vi "All Verifies With Labels.vi"   [LabVIEW 2020, in "Caraya Extension Tests.lvclass"]
uses:
  Caraya Extension Tests.lvclass
  Source/Approval Tests/Options/Options.lvclass/Options.ctl
  Source/Approval Tests/Naming Data/Naming Data.lvclass/Naming Data.ctl
  Source/Approval Tests/Options/Options.lvclass
  Source/Approval Tests/Scrubber/Scrubber.lvclass
  Source/Approval Tests/Namer/Namer.lvclass
  Source/Approval Tests/Naming Data/Naming Data.lvclass
  Source/Approval Tests/Reporter/Reporter.lvclass
  Source/Approval Tests/Text Comparator/Text Comparator.lvclass
  870c6c77-fc99-4cce-8b97-a4330b55fadd.vi
  Source/Extensions/Caraya.Extension/Caraya.Extension.lvlib
  <vilib>/addons/_JKI Toolkits/Caraya/classes/Test/Test.lvclass
  f52be7d2-abca-4f6a-8aa8-cd22b4bd47f7.vi
  9461663a-62e6-4c7f-8db7-86399d0571fe.vi
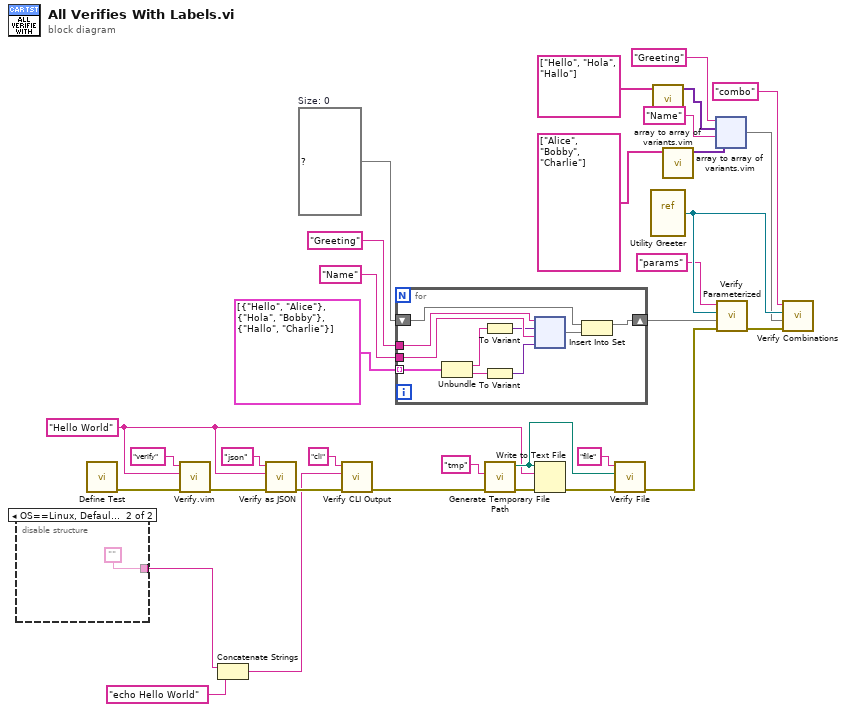
[diagram p0: block diagram]
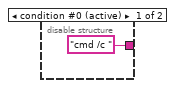
[diagram p2: hidden frame]
diagram:
  w24 = set{map{string, variant}} {}  # Size: 0
  w8 = "Hello World"
  n1 = disable-structure shown="OS==Linux, Default" {
    disable-tunnel: ["cmd /c " ""] -> w5
    frame condition #0 (active) {
    }
    frame condition #1 {
    }
  }
  n2 = call <vilib>:"Define Test.vi"() -> ("error out"=w31:errorcluster)  [unwired: 10 in, 1 out]
  n3 = call "Verify.vim"("error in"=w31, "Test Data"=w8, "Label"="verify") -> ("error out"=w33:errorcluster)  [unwired: 7 in, 1 out]
  n4 = Concatenate Strings(w5, "echo Hello World" ("string")) -> (w6:string)
  n5 = call "Verify as JSON.vi"("error in"=w33, "Anything"=w8, "Label"="json") -> ("error out"=w32:errorcluster)  [unwired: 7 in, 1 out]
  n6 = call "Verify CLI Output.vi"("error in"=w32, "command line"=w6, "Label"="cli") -> ("error out"=w28:errorcluster)  [unwired: 7 in, 1 out]
  n7 = for {
    tunnel: "Greeting" -> [w45]
    tunnel: cluster{string, string}[] [{"Hello", "Alice"}, {"Hola", "Bobby"}, {"Hallo", "Charlie"}] -> [w43] mode=indexing
    tunnel: "Name" -> [w44]
    shift-right: [w37] -> w25
    shift-left: w24 -> [w36]
    n8 = Unbundle(w43) -> (w42:string, w41:string)
    n9 = To Variant(anything=w42) -> (Variant=w39:variant)
    n10 = To Variant(anything=w41) -> (Variant=w38:variant)
    n11 = node ("Build Map")(w45, w39, w44, w38) -> (w40:map{string, variant})
    n12 = Insert Into Set(10:w40, 11:w36) -> (3:w37:set{map{string, variant}})  [unwired: 1 out]
  }
  n13 = call <vilib>:"Generate Temporary File Path.vi"("error in (no error)"=w28, "Temporary File Extension (tmp)"="tmp") -> ("error out"=w27:errorcluster, "Unique Temporary File Path"=w9:path)  [unwired: 8 in]
  n14 = Write to Text File(file (use dialog)=w9, text=w8, error in=w27) -> (error out=w26:errorcluster)  [unwired: 1 in, 2 out]
  n15 = call "Verify File.vi"("error in"=w26, "path to file"=w9, "Label"="file") -> ("error out"=w30:errorcluster)  [unwired: 7 in, 1 out]
  n16 = vi-ref "Utility Greeter.vi"() -> (w20:refnum<vi>)
  n17 = call "array to array of variants.vim"("Array in"=string[] ["Hello", "Hola", "Hallo"]) -> ("Array out"=w3:variant[])  [unwired: 10 in]
  n18 = call "array to array of variants.vim"("Array in"=string[] ["Alice", "Bobby", "Charlie"]) -> ("Array out"=w1:variant[])  [unwired: 10 in]
  n19 = node ("Build Map")("Greeting" ("key"), w3, "Name" ("key"), w1) -> (w19:map{string, variant[]})
  n20 = call "Verify Parameterized.vi"("error in"=w30, "ctl label -> value var"=w25, "VI Refnum"=w20, "Label"="params") -> ("error out"=w29:errorcluster)  [unwired: 6 in, 1 out]
  n21 = call "Verify Combinations.vi"("error in"=w29, "ctl label -> value var[]"=w19, "VI Refnum"=w20, "Label"="combo") -> ()  [unwired: 6 in, 2 out]
